vi "Polling Core.vi"(8 "Error In":errorcluster, 11 "BNT_DAQmx_MCSV-Ctr2Freq in":refnum<class "BNT_DAQmx-MCSV-Ctr2Freq.lvclass">) -> (0 "Error Out":errorcluster, 3 "BNT_DAQmx_MCSV-Ctr2Freq out":refnum<class "BNT_DAQmx-MCSV-Ctr2Freq.lvclass">)   [LabVIEW 2016, in "BNT_DAQmx.lvlib" / "BNT_DAQmx-MCSV-Ctr2Freq.lvclass"]
uses:
  BNT_DAQmx-MCSV-Ctr2Freq.lvclass
  C:/User/Brand/LVP/BNT/EQCR/Packages/BNT_DAQmx/BNT_DAQmx-MCSV/BNT_DAQmx-MCSV.lvclass
  BNT_DAQmx-MCSV/BNT_DAQmx-MCSV.lvclass/BNT_DAQmx-MCSV.ctl
  BNT_DAQmx-MCSV-Ctr2Freq.lvclass/BNT_DAQmx-MCSV-Ctr2Freq.ctl
  CSPP_Core/Classes/CS++ProcessVariables/PVConnection/PVConnection.lvclass/PVConnection.ctl
  CSPP_Core/Classes/CS++ProcessVariables/ProcessVariable/PV.lvclass/PV.ctl
  CSPP_Core/Classes/CS++ProcessVariables/ProcessVariable/Write Data.vi
  CSPP_Core/Classes/CS++ProcessVariables/ProcessVariable/Write Error.vi
  CSPP_Core/Classes/CS++ProcessVariables/ProcessVariable/Write Quality.vi
  CSPP_Core/Classes/CS++ProcessVariables/ProcessVariable/Write status.vi
  CSPP_Core/Classes/CS++ProcessVariables/ProcessVariable/Write Timestamp.vi
  CSPP_Core/Classes/CS++ProcessVariables/ProcessVariable/PV.lvclass
  BNT_DAQmx-MCSV/BNT_DAQmx-MCSV.lvclass
  CSPP_Core/Classes/CS++ProcessVariables/PVConnection/PVConnection.lvclass
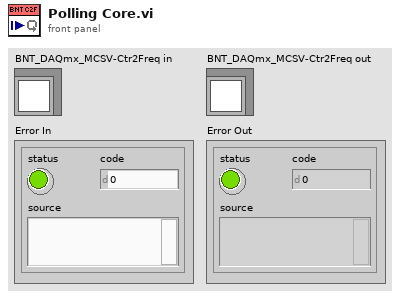
[diagram p1: front panel]
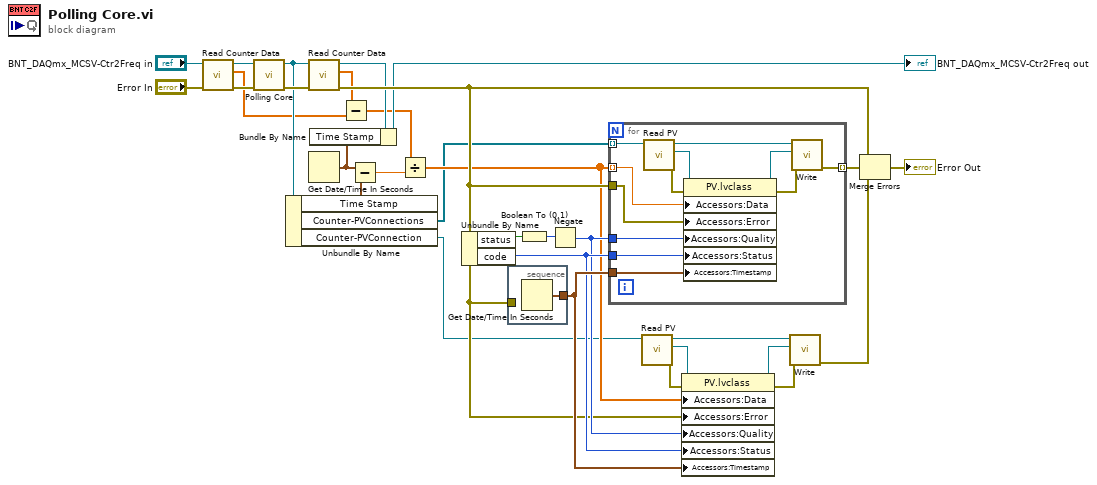
[diagram p0: block diagram]
diagram:
  n1 = call "Read Counter Data.vi"("error in (no error)"="Error In", "BNT_DAQmx-MCSV in"="BNT_DAQmx_MCSV-Ctr2Freq in") -> ("error out"=w4:errorcluster, "Counter Data"=w3:dbl[], "BNT_DAQmx-MCSV out"=w6:refnum<class "BNT_DAQmx-MCSV-Ctr2Freq.lvclass">)  [unwired: 7 in]
  n2 = call-parent "Polling Core.vi"("Error In"=w4, "BNT_DAQmx-MCSV in"=w6) -> ("Error Out"=w31:errorcluster, "BNT_DAQmx-MCSV out"=w30:refnum<class "BNT_DAQmx-MCSV-Ctr2Freq.lvclass">)  [unwired: 8 in]
  n3 = Unbundle By Name(w30) -> ("Time Stamp"=w29:timestamp, "Counter-PVConnections"=w13:refnum<class "PVConnection.lvclass">[], "Counter-PVConnection"=w12:refnum<class "PVConnection.lvclass">)
  n4 = call "Read Counter Data.vi"("error in (no error)"=w31, "BNT_DAQmx-MCSV in"=w30) -> ("error out"=w15:errorcluster, "Counter Data"=w2:dbl[], "BNT_DAQmx-MCSV out"=w10:refnum<class "BNT_DAQmx-MCSV-Ctr2Freq.lvclass">)  [unwired: 7 in]
  n5 = Get Date/Time In Seconds() -> (seconds since 1Jan1904=w11:timestamp)
  n6 = Bundle By Name(cluster=w10, "Time Stamp"=w11) -> (→"BNT_DAQmx_MCSV-Ctr2Freq out":refnum<class "BNT_DAQmx-MCSV-Ctr2Freq.lvclass">)
  n7 = Subtract(x=w2, y=w3) -> (x-y=w1:dbl[])
  n8 = Subtract(x=w11, y=w29) -> (x-y=w28:dbl)
  n9 = Divide(x=w1, y=w28) -> (x/y=w14:dbl[])
  n10 = Unbundle By Name(w15) -> ("status"=w17:bool, "code"=w25:i32)
  n11 = stacked-sequence {
    tunnel: [w32] -> w26
    tunnel: w15 -> [_]
    frame #0 {
      n12 = Get Date/Time In Seconds() -> (seconds since 1Jan1904=w32:timestamp)
    }
  }
  n13 = Boolean To (0,1)(Boolean=w17) -> (0, 1=w16:i16)
  n14 = Negate(x=w16) -> (-x=w24:i16)
  n15 = for {
    tunnel: w13 -> [w36] mode=indexing
    tunnel: w14 -> [w44] mode=indexing
    tunnel: w15 -> [w43]
    tunnel: [w40] -> w18 mode=indexing
    tunnel: w24 -> [w39]
    tunnel: w25 -> [w38]
    tunnel: w26 -> [w37]
    n16 = call "Read PV.vi"("PVConnection in"=w36) -> ("error out"=w33:errorcluster, "PV"=w34:refnum<class "PV.lvclass">, "PVConnection out"=w35:refnum<class "PVConnection.lvclass">)  [unwired: 8 in]
    n17 = property class="PV.lvclass"(reference=w34, error in=w33, "Accessors:Data"=w44, "Accessors:Error"=w43, "Accessors:Quality"=w39, "Accessors:Status"=w38, "Accessors:Timestamp"=w37) -> (reference out=w42:refnum<class "PV.lvclass">, error out=w41:errorcluster)
    n18 = call "Write.vi"("error in (no error)"=w41, "PV"=w42, "PVConnection in"=w35) -> ("error out"=w40:errorcluster)  [unwired: 7 in, 1 out]
  }
  n19 = call "Read PV.vi"("PVConnection in"=w12) -> ("error out"=w19:errorcluster, "PV"=w20:refnum<class "PV.lvclass">, "PVConnection out"=w21:refnum<class "PVConnection.lvclass">)  [unwired: 8 in]
  n20 = property class="PV.lvclass"(reference=w20, error in=w19, "Accessors:Data"=w14, "Accessors:Error"=w15, "Accessors:Quality"=w24, "Accessors:Status"=w25, "Accessors:Timestamp"=w26) -> (reference out=w23:refnum<class "PV.lvclass">, error out=w22:errorcluster)
  n21 = call "Write.vi"("error in (no error)"=w22, "PV"=w23, "PVConnection in"=w21) -> ("error out"=w27:errorcluster)  [unwired: 7 in, 1 out]
  n22 = Merge Errors(w15, w18, w27) -> (→"Error Out":errorcluster)
